vi "子界面-查看某框和报告生成-第2版.vi"(0 "框号":dbl format="%#_13g", 1 "框组":T3(array[cluster]), 3 "反射图原始路径":path, 5 "预先配置的灰度阈值":dbl, 6 "穿透图原始路径":path, 7 "部位信息":string[](array[string])=["", "34.500000", "32.500000", "1121", "34", "54.955926", "分层类", "不合格", ""], 12 "产品规格":cluster{"产品长度（周长）（mm）":dbl, "产品宽度（母线长）（mm）":dbl}) -> (14 "弥散类检测结果":string[][](table), 19 "分层类检测结果":string[][](table))   [LabVIEW 2018]
uses:
  <vilib>/vision/NI_Vision_Development_Module.lvlib
panel:
  out "弥散缺陷个数":i32
  out "分层缺陷个数":i32
  out "?":dbl[][](array[numeric])
  out "合格？ 弥散类":string="fencengThreshold"
  out "合格？分层类":string="fencengThreshold"
  in  "stop":bool caption="停止"
  out "?":T1(plugin-control)
  out "Threshold Image":T1(plugin-control)
  out "Threshold Image":T1(plugin-control)
  out "Threshold Image":T1(plugin-control)
  out "反射图ROI的最大灰度值":sgl
  in  "灰度阈值设置":cluster{"下限":dbl, "下限":dbl}(slide)={"下限"=0.0, "下限"=65.10638427734375} scale=0.0..255.0
  in  "Tab Control":T2
  out "穿透ROI":T1(plugin-control)
  out "Threshold Image":T1(plugin-control)
  out "?":T1(plugin-control)
  out "?":T1(plugin-control)
  out "Threshold Image":T1(plugin-control)
  out "Threshold Image":T1(plugin-control)
  out "弥散测量结果":dbl[][](array[numeric]) format="%.2f"
  in  "分隔符（'\\'代码显示）":string="\t"
  in  "格式字符串":string="%f"
  out "?":string
  out "面积 (pixels)":i32
  in  "格式字符串 2":string="%f"
  in  "分隔符（'\\'代码显示）":string="\t"
  out "分层测量结果":dbl[][](array[numeric]) format="%.2f"
  out "缺陷分类的临界值":sgl format="%#.3f"
  # "所选区域信息"
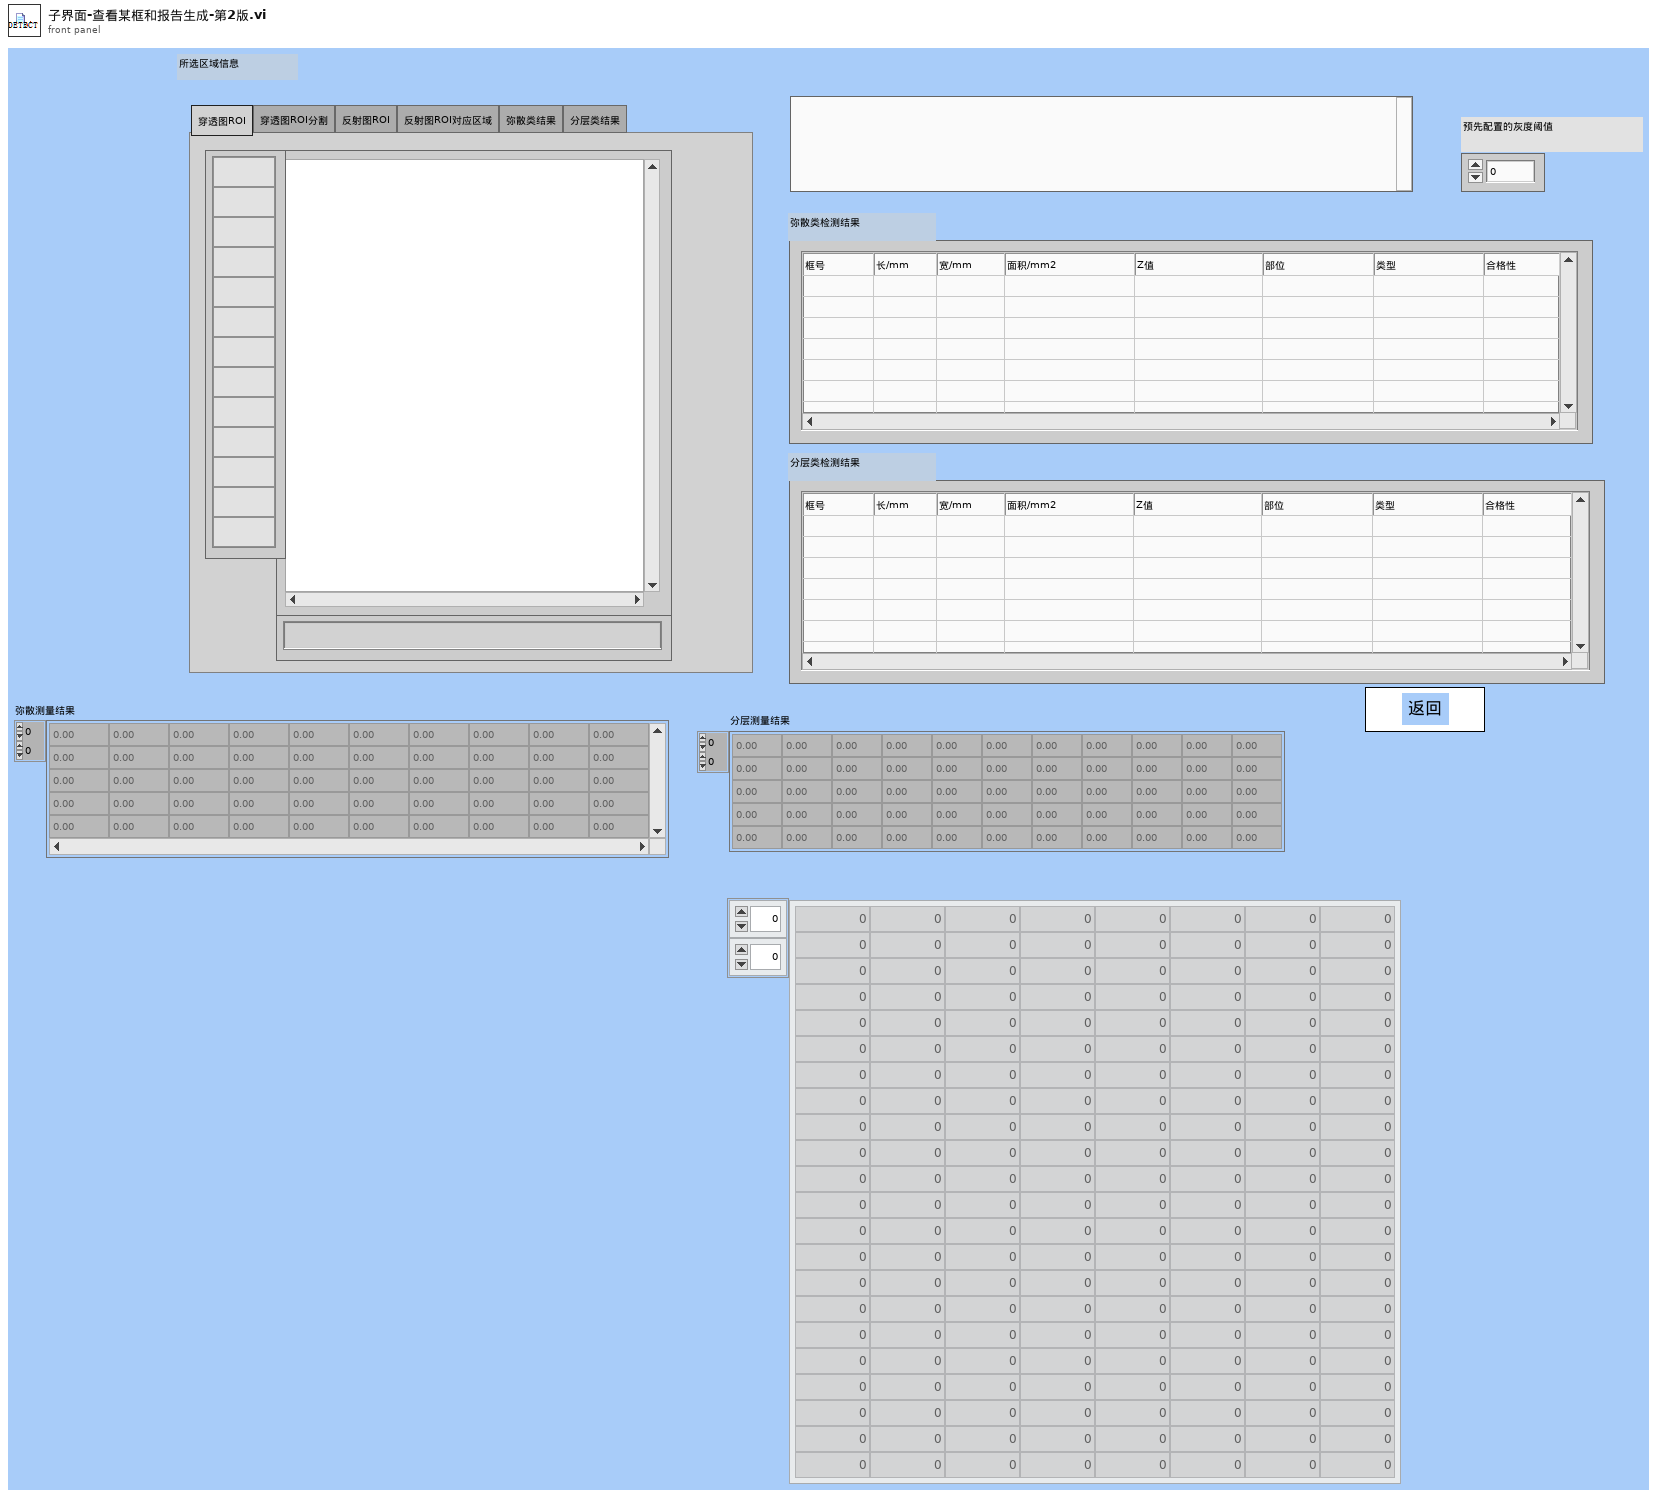
[diagram p1: front panel]
types:
  T1 = typedef "IMAQ Image.ctl" = refnum<image>
  T2 = typedef "控件 1.ctl" = enum32{"穿透图ROI", "穿透图ROI分割", "反射图ROI", "反射图ROI对应区域", "弥散类结果", "分层类结果"}
  T3 = cluster{"Global Rectangle":i32[], "Contours":cluster{"Contour Type":u32, "ROI Type":u32, "Points":i32[]}[]}[]
  T4 = typedef "Image Type" = u32
  T5 = typedef "Particle Parameters" = i32
  T6 = cluster{"Measurement Parameter":T5, "Range Lower Value":dbl, "Range Upper Value":dbl, "Range":bool, "Measurement Type":bool}[]
  T7 = cluster{"Global Rectangle":i32[], "Contours":cluster{"Contour Type":u32, "ROI Type":u32, "Points":i32[]}[]}
  T8 = cluster{"histogram":u32[], "Minimal Value":sgl, "Maximal Value":sgl, "Starting Value":sgl, "Interval Width":sgl, "Mean Value":sgl, "Standard  Variation":sgl, "Area (pixels)":i32}
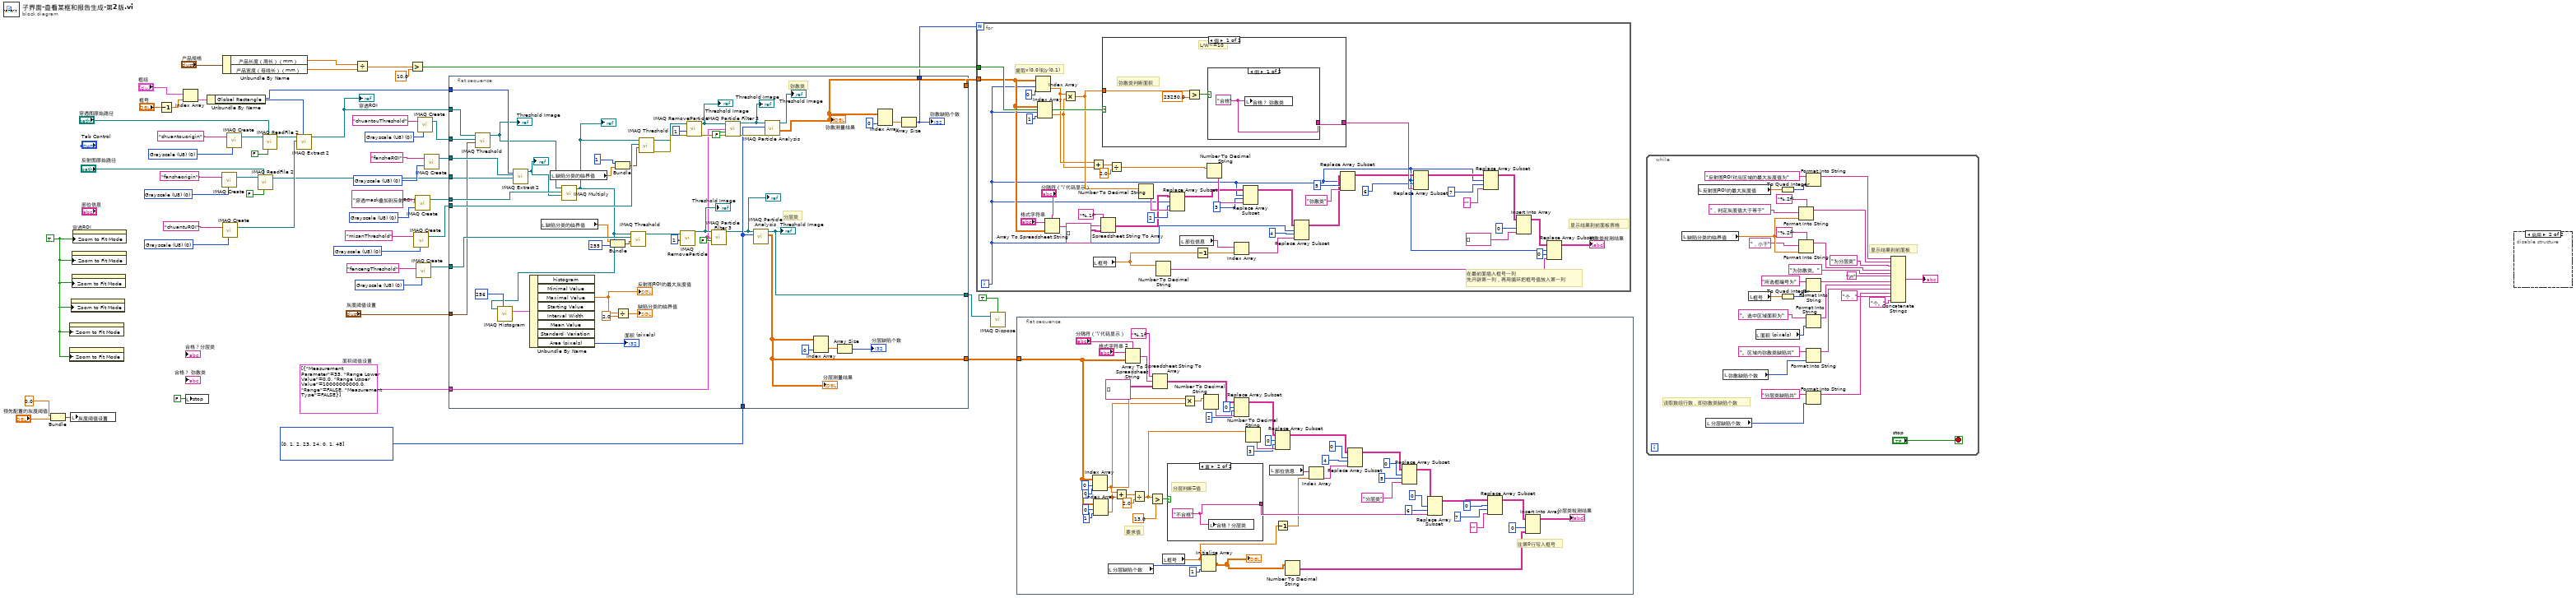
[diagram p0: block diagram]
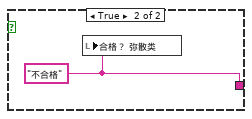
[diagram p2: hidden frame]
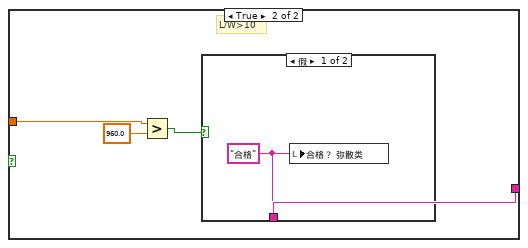
[diagram p3: hidden frame]
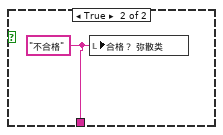
[diagram p4: hidden frame]
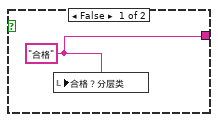
[diagram p5: hidden frame]
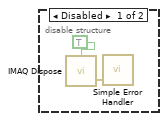
[diagram p6: hidden frame]
diagram:
  w3 = T4 0 items=["Grayscale (U8)", "Grayscale (I16)", "Grayscale (SGL)", "Complex (CSG)", "RGB (U32)", "HSL (U32)", "RGB (U64)", "Grayscale (U16)"] ("Image Type")
  w4 = T4 0 items=["Grayscale (U8)", "Grayscale (I16)", "Grayscale (SGL)", "Complex (CSG)", "RGB (U32)", "HSL (U32)", "RGB (U64)", "Grayscale (U16)"] ("Image Type")
  w5 = T4 0 items=["Grayscale (U8)", "Grayscale (I16)", "Grayscale (SGL)", "Complex (CSG)", "RGB (U32)", "HSL (U32)", "RGB (U64)", "Grayscale (U16)"] ("Image Type")
  w10 = T4 0 items=["Grayscale (U8)", "Grayscale (I16)", "Grayscale (SGL)", "Complex (CSG)", "RGB (U32)", "HSL (U32)", "RGB (U64)", "Grayscale (U16)"] ("Image Type")
  w15 = T4 0 items=["Grayscale (U8)", "Grayscale (I16)", "Grayscale (SGL)", "Complex (CSG)", "RGB (U32)", "HSL (U32)", "RGB (U64)", "Grayscale (U16)"] ("Image Type")
  w29 = i32[] [0, 1, 2, 23, 24, 0, 1, 48] items=["Bounding Rect Width", "Bounding Rect Height", "Area"] ("Pixel Measurements")
  w30 = T6 [{"Measurement Parameter"=35, "Range Lower Value"=0.0, "Range Upper Value"=10000000000.0, "Range"=FALSE, "Measurement Type"=FALSE}]  # 面积阈值设置
  w37 = T4 0 items=["Grayscale (U8)", "Grayscale (I16)", "Grayscale (SGL)", "Complex (CSG)", "RGB (U32)", "HSL (U32)", "RGB (U64)", "Grayscale (U16)"] ("Image Type")
  w41 = T4 0 items=["Grayscale (U8)", "Grayscale (I16)", "Grayscale (SGL)", "Complex (CSG)", "RGB (U32)", "HSL (U32)", "RGB (U64)", "Grayscale (U16)"] ("Image Type")
  w46 = T4 0 items=["Grayscale (U8)", "Grayscale (I16)", "Grayscale (SGL)", "Complex (CSG)", "RGB (U32)", "HSL (U32)", "RGB (U64)", "Grayscale (U16)"] ("Image Type")
  w55 = TRUE ("Zoom to Fit Mode")
  n1 = Bundle(0.0, "预先配置的灰度阈值"="预先配置的灰度阈值") -> (w53:cluster{dbl, "预先配置的灰度阈值":dbl})  [unwired: 1 in]
  n2 = property class="ImageControl"("Zoom to Fit Mode"=w55) -> ()  [unwired: 2 in, 2 out]
  n3 = property class="ImageControl"("Zoom to Fit Mode"=w55) -> ()  [unwired: 2 in, 2 out]
  n4 = local write "灰度阈值设置"(w53) -> ()
  n5 = property class="ImageControl"("Zoom to Fit Mode"=w55) -> ()  [unwired: 2 in, 2 out]
  n6 = property class="ImageControl"("Zoom to Fit Mode"=w55) -> ()  [unwired: 2 in, 2 out]
  n7 = property class="ImageControl"("Zoom to Fit Mode"=w55) -> ()  [unwired: 2 in, 2 out]
  n8 = property on="穿透ROI" class="ImageControl"("Zoom to Fit Mode"=w55) -> ()  [unwired: 2 in, 2 out]
  n9 = Decrement(x="框号") -> (x-1=w48:dbl)
  n10 = Index Array(array="框组", index=w48) -> (element=w49:T7)
  n11 = local write "stop"(FALSE ("stop")) -> ()
  n12 = Unbundle By Name(w49) -> ("Global Rectangle"=w32:i32[])
  n13 = call "IMAQ Create"("Image Name"="fansheorigin", "Image Type"=w10) -> ("New Image"=w9:T1)  [unwired: 3 in, 1 out]
  n14 = call "IMAQ Create"("Image Name"="chuantuROI", "Image Type"=w15) -> ("New Image"=w14:T1)  [unwired: 3 in, 1 out]
  n15 = Unbundle By Name("产品规格") -> ("产品长度（周长）（mm）"=w25:dbl, "产品宽度（母线长）（mm）"=w24:dbl)
  n16 = call "IMAQ Create"("Image Name"="chuantouorigin", "Image Type"=w46) -> ("New Image"=w17:T1)  [unwired: 3 in, 1 out]
  n17 = call "IMAQ ReadFile 2"("Use File Path Image Type"=FALSE, "File Path"="反射图原始路径", "Image"=w9) -> ("Image Out"=w6:T1)  [unwired: 4 in, 4 out]
  n18 = call "IMAQ ReadFile 2"("Use File Path Image Type"=FALSE, "File Path"="穿透图原始路径", "Image"=w17) -> ("Image Out"=w18:T1)  [unwired: 4 in, 4 out]
  n19 = call "IMAQ Extract 2"("Optional Rectangle"=w32, "Image Dst"=w14, "Image Src"=w18) -> ("Image Dst Out"=w39:T1)  [unwired: 7 in, 1 out]
  "穿透ROI" <- w39
  n20 = Divide(x=w25, y=w24) -> (x/y=w28:dbl)
  n21 = Greater?(x=w28, y=10.0) -> (0:w22:bool)
  n22 = call "IMAQ Create"("Image Name"="misanThreshold", "Image Type"=w3) -> ("New Image"=w35:T1)  [unwired: 3 in, 1 out]
  n23 = call "IMAQ Create"("Image Name"="穿透mask叠加到反射ROI上", "Image Type"=w37) -> ("New Image"=w36:T1)  [unwired: 3 in, 1 out]
  n24 = call "IMAQ Create"("Image Name"="fencengThreshold", "Image Type"=w4) -> ("New Image"=w33:T1)  [unwired: 3 in, 1 out]
  n25 = call "IMAQ Create"("Image Name"="chuantouThreshold", "Image Type"=w5) -> ("New Image"=w43:T1)  [unwired: 3 in, 1 out]
  n26 = call "IMAQ Create"("Image Name"="fansheROI", "Image Type"=w41) -> ("New Image"=w40:T1)  [unwired: 3 in, 1 out]
  n27 = flat-sequence {
    tunnel: w43 -> [w104]
    tunnel: w40 -> [w103]
    tunnel: w39 -> [w102]
    tunnel: w36 -> [w101]
    tunnel: w35 -> [w100]
    tunnel: w33 -> [w99]
    tunnel: w32 -> [w98]
    tunnel: w30 -> [w70]
    tunnel: w29 -> [w69]
    tunnel: [w68] -> w23
    tunnel: [w67] -> w21
    tunnel: [w61] -> w20
    tunnel: [w58] -> w1
    tunnel: "灰度阈值设置" -> [w57]
    tunnel: w6 -> [w56]
    frame #0 {
      # "弥散类"
      # "分层类"
      n28 = call "IMAQ Threshold"("Range"=w57, "Image Dst"=w104, "Image Src"=w102) -> ("Image Dst Out"=w88:T1)  [unwired: 3 in, 5 out]
      "Threshold Image" <- w88
      n29 = call "IMAQ Extract 2"("Optional Rectangle"=w98, "Image Dst"=w103, "Image Src"=w56) -> ("Image Dst Out"=w87:T1)  [unwired: 7 in, 1 out]
      "?" <- w87
      n30 = local read "缺陷分类的临界值"() -> (w75:sgl)
      n31 = local read "缺陷分类的临界值"() -> (w82:sgl)
      n32 = call "IMAQ Multiply"("Image Src A"=w88, "Image Dst"=w101, "Image Src B"=w87) -> ("Image Dst Out"=w78:T1)  [unwired: 4 in, 1 out]
      "?" <- w78
      n33 = call "IMAQ Histogram"("Number of Classes"=256, "Image"=w78) -> ("Histogram Report"=w91:T8)  [unwired: 8 in, 1 out]
      n34 = Unbundle By Name(w91) -> ("Maximal Value"=w86:sgl, "Area (pixels)"=→"面积 (pixels)":i32)  [unwired: 6 out]
      "反射图ROI的最大灰度值" <- w86
      n35 = Bundle("缺陷分类的临界值"=w75, 255) -> (w77:cluster{"缺陷分类的临界值":sgl, i32})  [unwired: 1 in]
      n36 = Bundle(1, "缺陷分类的临界值"=w82) -> (w81:cluster{i32, "缺陷分类的临界值":sgl})  [unwired: 1 in]
      n37 = Divide(x=w86, y=sgl 2.0) -> (x/y=→"缺陷分类的临界值":sgl)
      n38 = call "IMAQ Threshold"("Range"=w77, "Image Dst"=w99, "Image Src"=w78) -> ("Image Dst Out"=w74:T1)  [unwired: 3 in, 5 out]
      n39 = call "IMAQ Threshold"("Range"=w81, "Image Dst"=w100, "Image Src"=w78) -> ("error out"=w95:errorcluster, "Image Dst Out"=w92:T1)  [unwired: 3 in, 4 out]
      n40 = call "IMAQ RemoveParticle"("Number of Erosion"=1, "Image Src"=w74) -> ("Image Dst Out"=w71:T1)  [unwired: 8 in, 1 out]
      "Threshold Image" <- w71
      n41 = call "IMAQ RemoveParticle"("error in (no error)"=w95, "Number of Erosion"=1, "Image Src"=w92) -> ("error out"=w94:errorcluster, "Image Dst Out"=w80:T1)  [unwired: 7 in]
      "Threshold Image" <- w80
      n42 = call "IMAQ Particle Filter 3"("Image Src"=w71, "Selection Values"=w70, "Keep/Remove Particles (F)"=FALSE) -> ("Image Dst Out"=w60:T1)  [unwired: 10 in, 2 out]
      "?" <- w60
      n43 = call "IMAQ Particle Filter 3"("Image Src"=w80, "Selection Values"=w70, "Keep/Remove Particles (F)"=FALSE, "error in (no error)"=w94) -> ("Image Dst Out"=w79:T1, "error out"=w93:errorcluster)  [unwired: 9 in, 1 out]
      "Threshold Image" <- w79
      n44 = call "IMAQ Particle Analysis"("Pixel Measurements"=w69, "Image"=w60) -> ("Particle Measurements (Pixels)"=w68:dbl[][], "Image Out (duplicate)"=w58:T1)  [unwired: 4 in, 4 out]
      "Threshold Image" <- w58
      "分层测量结果" <- w68
      n45 = call "IMAQ Particle Analysis"("error in (no error)"=w93, "Pixel Measurements"=w69, "Image"=w79) -> ("Particle Measurements (Real-World)"=w67:dbl[][], "Image Out (duplicate)"=→"Threshold Image":T1)  [unwired: 3 in, 4 out]
      "弥散测量结果" <- w67
      n46 = Index Array(array=w68, index (col)=0 ("禁用的索引 (列)")) -> (element=w65:dbl[])  [unwired: 1 in]
      n47 = Array Size(array=w65) -> (size(s)=→"分层缺陷个数":i32)
      n48 = Index Array(array=w67, index (col)=0 ("禁用的索引 (列)")) -> (element=w63:dbl[])  [unwired: 1 in]
      n49 = Array Size(array=w63) -> (size(s)=w61:i32)
      "弥散缺陷个数" <- w61
    }
  }
  n50 = for {
    N: w20 -> [_]
    tunnel: w22 -> [w148]
    tunnel: w21 -> [w147]
    i -> [w108]
    # "在最前面插入框号一列\n先开辟第一列，再用循环把框号值放入第一列"
    # "提取x(0,0)和y(0,1)"
    # "显示结果到前面板表格"
    n51 = Index Array(array=w147, index (row)=w108, index (col)=0 ("禁用的索引 (列)")) -> (element=w131:dbl)
    n52 = Index Array(array=w147, index (row)=w108, index (col)=1 ("禁用的索引 (列)")) -> (element=w130:dbl)
    n53 = Array To Spreadsheet String(delimiter (Tab)="分隔符（'\\'代码显示）", array=w147, 3:"格式字符串") -> (spreadsheet string=w145:string)
    n54 = Multiply(x=w131, y=w130) -> (x*y=w134:dbl)
    n55 = Add(x=w131, y=w130) -> (x+y=w133:dbl)
    n56 = local read "框号"() -> (w112:dbl)
    n57 = Spreadsheet String To Array(format string="%.1f", spreadsheet string=w145, array type (2D Dbl)=string[][] [] ("Array")) -> (array=w122:string[][])  [unwired: 1 in]
    n58 = case shown="假" w148 {
      tunnel: w134 -> [w151 w158]
      tunnel: [w149 w155] -> w146
      frame False {
        # "弥散类判断面积"
        # "L/W<=10"
        n59 = Greater?(x=w151, y=23250.0) -> (0:w150:bool)
        n60 = case shown="假" w150 {
          tunnel: [w153 w154] -> w149
          frame False {
            w153 = "合格" ("合格？")
            n61 = local write "合格？ 弥散类"(w153) -> ()
          }
          frame True {
            w154 = "不合格" ("合格？")
            n62 = local write "合格？ 弥散类"(w154) -> ()
          }
        }
      }
      frame True {
        # "L/W>10"
        n63 = Greater?(x=w158, y=960.0) -> (0:w156:bool)
        n64 = case shown="假" w156 {
          tunnel: [w159 w160] -> w155
          frame False {
            w159 = "合格" ("合格？")
            n65 = local write "合格？ 弥散类"(w159) -> ()
          }
          frame True {
            w160 = "不合格" ("合格？")
            n66 = local write "合格？ 弥散类"(w160) -> ()
          }
        }
      }
    }
    n67 = Divide(x=w133, y=2.0) -> (x/y=w127:dbl)
    n68 = Number To Decimal String(number=w134) -> (decimal integer string=w136:string)  [unwired: 1 in]
    n69 = Number To Decimal String(number=w112) -> (decimal integer string=w106:string)  [unwired: 1 in]
    n70 = Replace Array Subset(array=w122, new element=w136, index (row)=w108, index (col)=2 ("禁用的索引 (列)")) -> (w121:string[][])
    n71 = local read "部位信息"() -> (w117:string[])
    n72 = Decrement(x=w112) -> (x-1=w116:dbl)
    n73 = Number To Decimal String(number=w127) -> (decimal integer string=w129:string)  [unwired: 1 in]
    n74 = Index Array(array=w117, index=w116) -> (element=w115:string)
    n75 = Replace Array Subset(array=w121, new element=w129, index (row)=w108, index (col)=3 ("禁用的索引 (列)")) -> (w114:string[][])
    n76 = Replace Array Subset(array=w114, new element=w115, index (row)=w108, index (col)=4 ("禁用的索引 (列)")) -> (w113:string[][])
    n77 = Replace Array Subset(array=w113, new element="弥散类" ("新元素/子数组"), index (row)=w108, index (col)=5 ("禁用的索引 (列)")) -> (w120:string[][])
    n78 = Replace Array Subset(array=w120, new element=w146, index (row)=w108, index (col)=6 ("禁用的索引 (列)")) -> (w119:string[][])
    n79 = Replace Array Subset(array=w119, new element="" ("新元素/子数组"), index (row)=w108, index (col)=7 ("禁用的索引 (列)")) -> (w111:string[][])
    n80 = Insert Into Array(array=w111, index (col)=0 ("禁用的索引 (列)"), new element=string[] [] ("新元素/子数组")) -> (w109:string[][])  [unwired: 1 in]
    n81 = Replace Array Subset(array=w109, new element=w106, index (row)=w108, index (col)=0 ("禁用的索引 (列)")) -> (→"弥散类检测结果":string[][])
  }
  n82 = call "IMAQ Dispose"("All Images? (No)"=TRUE, "Image"=w1) -> ()  [unwired: 4 in, 1 out]
  n83 = flat-sequence {
    tunnel: w23 -> [w212]
    frame #0 {
      # "往第0行写入框号"
      # "要求值"
      n84 = Index Array(array=w212, index (row)=0 ("索引 (行)"), index (col)=0 ("禁用的索引 (列)")) -> (element=w186:dbl)
      n85 = Index Array(array=w212, index (row)=0 ("索引 (行)"), index (col)=1 ("禁用的索引 (列)")) -> (element=w185:dbl)
      n86 = local read "分层缺陷个数"() -> (w210:i32)
      n87 = Add(x=w186, y=w185) -> (x+y=w206:dbl)
      n88 = Array To Spreadsheet String(delimiter (Tab)="分隔符（'\\'代码显示）", array=w212, 3:"格式字符串 2") -> (spreadsheet string=w205:string)
      n89 = Divide(x=w206, y=2.0) -> (x/y=w187:dbl)
      n90 = Greater?(x=w187, y=13.0) -> (0:w207:bool)
      n91 = Spreadsheet String To Array(format string="%.1f", spreadsheet string=w205, array type (2D Dbl)=string[][] [] ("Array")) -> (array=w180:string[][])  [unwired: 1 in]
      n92 = local read "框号"() -> (w164:dbl)
      n93 = case shown="真" w207 {
        tunnel: [w213 w214] -> w208
        frame False {
          w213 = "合格" ("合格？")
          n94 = local write "合格？分层类"(w213) -> ()
        }
        frame True {
          w214 = "不合格" ("合格？")
          # "分层判断Z值"
          n95 = local write "合格？分层类"(w214) -> ()
        }
      }
      n96 = Multiply(x=w186, y=w185) -> (x*y=w181:dbl)
      n97 = Initialize Array(w164, w210, 1 ("维数大小")) -> (w209:dbl[][])
      "?" <- w209
      n98 = Number To Decimal String(number=w181) -> (decimal integer string=w184:string)  [unwired: 1 in]
      n99 = Replace Array Subset(array=w180, new element=w184, index (row)=0 ("索引 (行)"), index (col)=2 ("禁用的索引 (列)")) -> (w171:string[][])
      n100 = Number To Decimal String(number=w187) -> (decimal integer string=w190:string)  [unwired: 1 in]
      n101 = local read "部位信息"() -> (w165:string[])
      n102 = Replace Array Subset(array=w171, new element=w190, index (row)=0 ("索引 (行)"), index (col)=3 ("禁用的索引 (列)")) -> (w162:string[][])
      n103 = Decrement(x=w164) -> (x-1=w163:dbl)
      n104 = Number To Decimal String(number=w209) -> (decimal integer string=w211:string[][])  [unwired: 1 in]
      n105 = Index Array(array=w165, index=w163) -> (element=w166:string)
      n106 = Replace Array Subset(array=w162, new element=w166, index (row)=0 ("索引 (行)"), index (col)=4 ("禁用的索引 (列)")) -> (w161:string[][])
      n107 = Replace Array Subset(array=w161, new element="分层类" ("新元素/子数组"), index (row)=0 ("索引 (行)"), index (col)=5 ("禁用的索引 (列)")) -> (w170:string[][])
      n108 = Replace Array Subset(array=w170, new element=w208, index (row)=0 ("索引 (行)"), index (col)=6 ("禁用的索引 (列)")) -> (w177:string[][])
      n109 = Replace Array Subset(array=w177, new element="" ("新元素/子数组"), index (row)=0 ("索引 (行)"), index (col)=7 ("禁用的索引 (列)")) -> (w175:string[][])
      n110 = Insert Into Array(array=w175, index (col)=0 ("禁用的索引 (列)"), new element=w211) -> (→"分层类检测结果":string[][])  [unwired: 1 in]
    }
  }
  n111 = while {
    stop <- "stop" stop-if-true
    # "显示结果到前面板"
    # "读取数组行数，即弥散类缺陷个数"
    n112 = local read "缺陷分类的临界值"() -> (w245:sgl)
    n113 = local read "反射图ROI的最大灰度值"() -> (w237:sgl)
    n114 = local read "分层缺陷个数"() -> (w216:i32)
    n115 = local read "弥散缺陷个数"() -> (w215:i32)
    n116 = local read "框号"() -> (w233:dbl)
    n117 = local read "面积 (pixels)"() -> (w236:i32)
    n118 = To Quad Integer(1:w237) -> (0:w238:i64)
    n119 = To Quad Integer(1:w233) -> (0:w234:i64)
    n120 = Format Into String(format string="%.2f" ("格式字符串"), initial string="，判定灰度值大于等于" ("初始字符串"), w245) -> (resulting string=w240:string)  [unwired: 1 in, 1 out]
    n121 = Format Into String(format string="%.2f" ("格式字符串"), initial string="，小于" ("初始字符串"), w245) -> (resulting string=w239:string)  [unwired: 1 in, 1 out]
    n122 = Format Into String(initial string="反射图ROI对应区域的最大灰度值为" ("初始字符串"), w238) -> (resulting string=w241:string)  [unwired: 2 in, 1 out]
    n123 = Format Into String(initial string="所选框编号为" ("初始字符串"), w234) -> (resulting string=w232:string)  [unwired: 2 in, 1 out]
    n124 = Format Into String(initial string="。选中区域面积为" ("字符串"), w236) -> (resulting string=w242:string)  [unwired: 2 in, 1 out]
    n125 = Format Into String(initial string="。区域内弥散类缺陷共" ("初始字符串"), w215) -> (resulting string=w243:string)  [unwired: 2 in, 1 out]
    n126 = Format Into String(initial string="分层类缺陷共" ("初始字符串"), w216) -> (resulting string=w244:string)  [unwired: 2 in, 1 out]
    n127 = Concatenate Strings(w241, w240, "为分层类" ("初始字符串"), w239, "为弥散类。" ("初始字符串"), "\n", w232, w242, w243, "个，" ("字符串"), w244, "个。" ("字符串")) -> (→"?":string)
  }
  n128 = disable-structure shown="启用" {
    frame Disabled {
      n129 = call "IMAQ Dispose"("All Images? (No)"=TRUE) -> ("error out"=w247:errorcluster)  [unwired: 5 in]
      n130 = call <vilib>:"Simple Error Handler.vi"("error in (no error)"=w247) -> ()  [unwired: 4 in, 5 out]
    }
    frame Enabled {
    }
  }
